vi "Get Audio Device Configuration.vi"(8 "error in (no error)":errorcluster, 11 "Audio Device Refnum In":T4) -> (0 "error out":errorcluster, 1 "Audio Device Advanced Config":T1, 2 "Audio Device Config":T2, 3 "Audio Device Refnum Out":T4)   [LabVIEW 2020, in "G-Audio.lvlib"]
doc: "Get information about the configured audio device."
uses:
  G-Audio.lvlib
  Controls/Audio Device Refnum.ctl
  Controls/Audio Device Config.ctl
  Controls/Audio Device Format.ctl
  Controls/Audio Device Advanced Config.ctl
  <vilib>/Utility/error.llb/Error Cluster From Error Code.vi
  lib/g_audio_32.dll
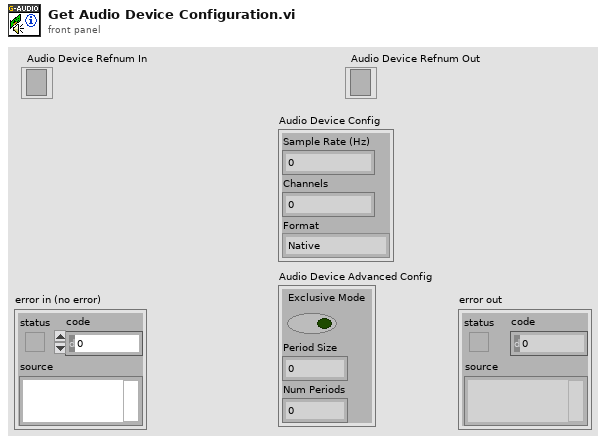
[diagram p1: front panel]
types:
  T1 = typedef "G-Audio.lvlib/Audio Device Advanced Config.ctl" = cluster{"Exclusive Mode":bool, "Period Size":u32, "Num Periods":u32}
  T2 = typedef "G-Audio.lvlib/Audio Device Config.ctl" = cluster{"Sample Rate (Hz)":u32, "Channels":u32, "Format":T3}
  T3 = typedef "G-Audio.lvlib/Audio Device Format.ctl" = enum16{"Native", "U8", "I16", "I32", "SGL"}
  T4 = typedef "G-Audio.lvlib/Audio Device Refnum.ctl" = refnum<file>
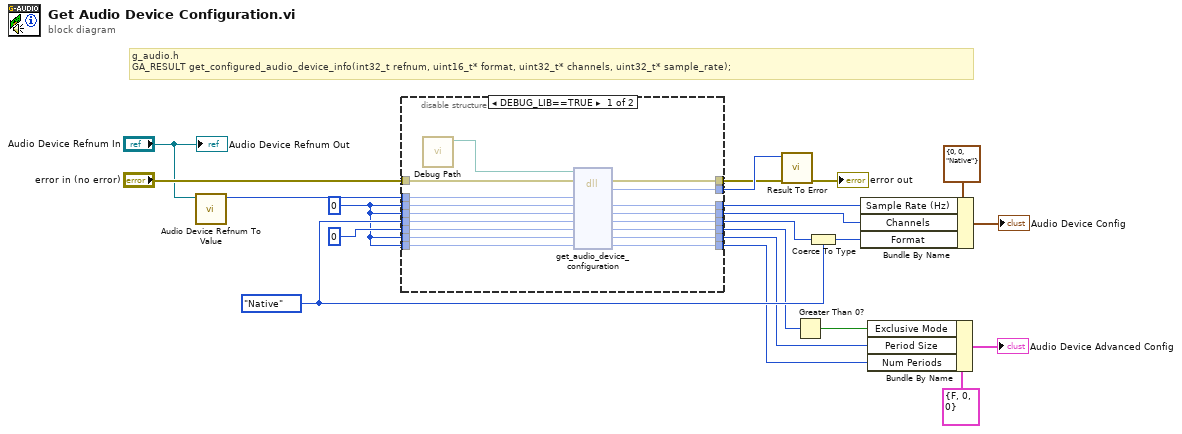
[diagram p0: block diagram]
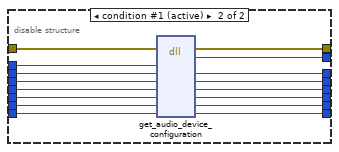
[diagram p2: hidden frame]
diagram:
  w17 = Audio_Device_Format."Native" ("Format")
  w4 = u32 0
  # "g_audio.h\nGA_RESULT get_configured_audio_device_info(int32_t refnum, uint16_t* format, uint32_t* channels, uint32_t* sample_rate);"
  n1 = call "Audio Device Refnum To Value.vi"("Audio Device Refnum"="Audio Device Refnum In") -> ("Refnum Value"=w7:i32)  [unwired: 10 in]
  n2 = disable-structure shown="DEBUG_LIB==TRUE" {
    disable-tunnel: "error in (no error)" -> [w38 w54]
    disable-tunnel: [w35 w51] -> w20
    disable-tunnel: [w37 w53] -> w19
    disable-tunnel: [w30 w47] -> w15
    disable-tunnel: w7 -> [w36 w52]
    disable-tunnel: w4 -> [w32 w49]
    disable-tunnel: w4 -> [w31 w48]
    disable-tunnel: [w29 w46] -> w12
    disable-tunnel: w17 -> [w33 w50]
    disable-tunnel: [w28 w45] -> w13
    disable-tunnel: u8 0 -> [w27 w44]
    disable-tunnel: [w26 w43] -> w10
    disable-tunnel: w4 -> [w25 w42]
    disable-tunnel: w4 -> [w24 w41]
    disable-tunnel: [w23 w40] -> w3
    disable-tunnel: [w22 w39] -> w2
    frame condition #0 {
      n3 = call "Debug Path.vi"() -> ("Debug Path"=w34:path)  [unwired: 11 in]
      n4 = dll-call lib="?" fn="get_audio_device_configuration"(path in=w34, error in=w38, "refnum"=w36, "sample_rate"=w32, "channels"=w31, "format"=w33, "exclusive_mode"=w27, "period_size"=w25, "num_periods"=w24) -> (error out=w37:errorcluster, "result"=w35:i32, "sample_rate"=w28:u32, "channels"=w29:u32, "format"=w30:u16, "exclusive_mode"=w26:u8, "period_size"=w23:u32, "num_periods"=w22:u32)  [unwired: 2 in, 1 out]
    }
    frame condition #1 (active) {
      n5 = dll-call lib="C:/github/dataflowg/g-audio/src/LabVIEW/G-Audio/lib/g_audio_*.*" fn="get_audio_device_configuration"(error in=w54, "refnum"=w52, "sample_rate"=w49, "channels"=w48, "format"=w50, "exclusive_mode"=w44, "period_size"=w42, "num_periods"=w41) -> (error out=w53:errorcluster, "result"=w51:i32, "sample_rate"=w45:u32, "channels"=w46:u32, "format"=w47:u16, "exclusive_mode"=w43:u8, "period_size"=w40:u32, "num_periods"=w39:u32)  [unwired: 3 in, 1 out]
    }
  }
  n6 = call "Result To Error.vi"("error in (no error)"=w19, "Result Code"=w20) -> ("error out"=→"error out":errorcluster)  [unwired: 9 in]
  n7 = Greater Than 0?(x=w10) -> (x > 0?=w5:bool)
  n8 = Coerce To Type(0:w15, 1:w17) -> (2:w14:T3)
  n9 = Bundle By Name(cluster=T2 {"Sample Rate (Hz)"=0, "Channels"=0, "Format"=enum."Native"} ("Audio Device Config"), "Sample Rate (Hz)"=w13, "Channels"=w12, "Format"=w14) -> (→"Audio Device Config":T2)
  n10 = Bundle By Name(cluster=T1 {"Exclusive Mode"=FALSE, "Period Size"=0, "Num Periods"=0} ("Audio Device Advanced Config"), "Exclusive Mode"=w5, "Period Size"=w3, "Num Periods"=w2) -> (→"Audio Device Advanced Config":T1)
  "Audio Device Refnum Out" <- "Audio Device Refnum In"
